vi "SOUR_POW_CORR_COLL_AVER_NTOL.vi"(0 "VISA IN":refnum<visa-resource-name>, 5 "error in":errorcluster, 7 "Settling Tolerance(dB)":dbl) -> (14 "VISA Out":refnum<visa-resource-name>, 19 "error out":errorcluster)   [LabVIEW 2018, in "PNA-X.lvlib"]
doc: "SOURce:POWer:CORRection:COLLect:AVERage:NTOLerance <num> \n(Read-Write) This command, along with SOUR:POW:CORR:COLL:AVER:COUNT, allows for \nsettling of the power sensor READINGS. \nEach power reading is averaged with the previous readings at each stimulus point. When the average \nmeets this nominal tolerance value or the max number of readings has been made, the average is \nreturned as the valid reading. \nThis setting is not necessary when using a PNA receiver (SOUR:POW:CORR:COLL REC) to make \nthe measurement. \nLearn more. \nParameters \n<num> Power measurement settling tolerance value in dB. Choose any number \nbetween 0 and 5. \nExamples SOUR:POW:CORR:COLL:AVER:NTOL .05 \nsource1:power2:correction:collect:average:ntolerance .003 \n1837\n\nQuery Syntax SOURce:POWer:CORRection:COLLect:AVERage:NTOLerance? \nReturn Type Numeric \nDefault .050 dBm \nSOURce<cnum>:POWer:CORRection:COLLect:DISPlay[:STATe] <ON | OFF> \n(Read-Write) Enables and disables the display of power readings on the PNA screen. Send this \ncommand BEFORE you begin a source power cal acquisition. After the source power cal data is \nacquired, this setting is reset to ON. \nParameters \n<cnum> Any existing channel number. If unspecified, value is set to 1 \n<ON|OFF> ON (1) Source power calibration dialog box is shown on the PNA screen. \nPower readings are plotted against the Tolerance value as limit lines. \nOFF (0) - Source power calibration dialog box is NOT shown on the PNA \nscreen. \nExamples SOUR:POW:CORR:COLL:DISP ON \nsource1:power2:correction:collect:display:state off \nQuery Syntax SOURce:POWer:CORRection:COLLect:DISPlay[:STATe]? \nReturn Type Boolean (1 = ON, 0 = OFF) \nDefault ON (1) \nSOURce<cnum>:POWer:CORRection:COLLect:FCHeck[:STATe] <ON | OFF> \n(Read-Write) Enables and disables frequency checking of source power cal acquisition sweeps. \nONLY use when you have more than one power sensor. \nParameters \n<cnum> Any existing channel number. If unspecified, value is set to 1 \n<ON|OFF> ON (1) turns source power cal frequency checking ON. A requested \nacquisition will only succeed for those frequency points which fall within a \nfrequency range specified for the power sensor being used. An acquisition will \npause in mid-sweep if the frequency is about to exceed the maximum \nfrequency limit specified for that sensor. When the sweep is paused in this \nmanner, a sensor connected to the other channel input of the power meter can \nbe connected to the measurement port in place of the previous sensor, and used \nto complete the sweep. However, the maximum frequency specified for the \n1838\n\nsecond sensor would need to be sufficient for the sweep to complete. \nFrequency limits are specified using the SOUR:POW:CORR:COLL:SEN \ncommand. \nOFF (0) - turns source power cal frequency checking OFF. An acquisition will \nuse just one power sensor for the entire sweep, regardless of frequency. \nExamples SOUR:POW:CORR:COLL:FCH ON \nsource1:power2:correction:collect:fcheck:state off \nQuery Syntax SOURce:POWer:CORRection:COLLect:FCHeck[:STATe]? \nReturn Type Boolean (1 = ON, 0 = OFF) \nDefault OFF (0)"
uses:
  PNA-X.lvlib
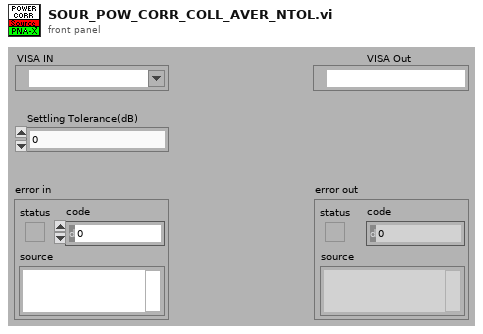
[diagram p1: front panel]
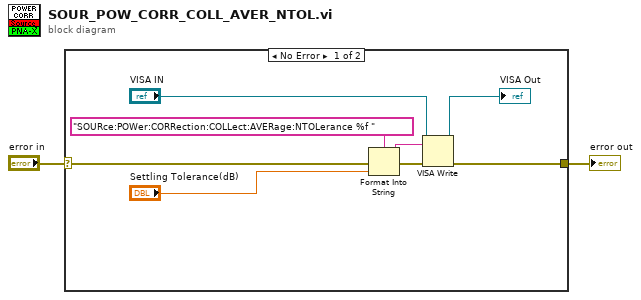
[diagram p0: block diagram]
diagram:
  n1 = case shown="No Error" "error in" {
    selector: "error in" -> [w10 w11]
    tunnel: [w5 w11] -> w1
    frame No Error {
      n2 = Format Into String(format string="SOURce:POWer:CORRection:COLLect:AVERage:NTOLerance %f " ("Cmdline"), error in=w10, "Settling Tolerance(dB)") -> (resulting string=w8:string, error out=w9:errorcluster)  [unwired: 1 in]
      n3 = VISA Write(VISA resource name="VISA IN", write buffer=w8, error in (no error)=w9) -> (VISA resource name out=→"VISA Out":refnum<visa-resource-name>, error out=w5:errorcluster)  [unwired: 1 out]
    }
    frame Error {
    }
  }
  "error out" <- w1
